vi "Create New File.vi"(8 "error in (no error)":errorcluster, 11 "[M] TDMS Save in":refnum<class "[M] TDMS Save.lvclass">) -> (0 "error out":errorcluster, 3 "[M] TDMS Save out":refnum<class "[M] TDMS Save.lvclass">)   [LabVIEW 2023, in "[M] TDMS Save.lvlib" / "[M] TDMS Save.lvclass"]
uses:
  [M] TDMS Save.lvclass
  [M] TDMS Save.lvclass/[M] TDMS Save.ctl
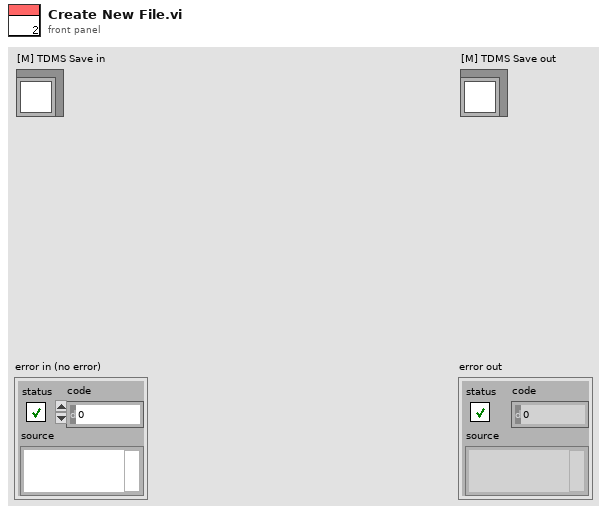
[diagram p1: front panel]
types:
  T1 = enum16{"open", "open or create", "create or replace", "create", "open (read-only)"}
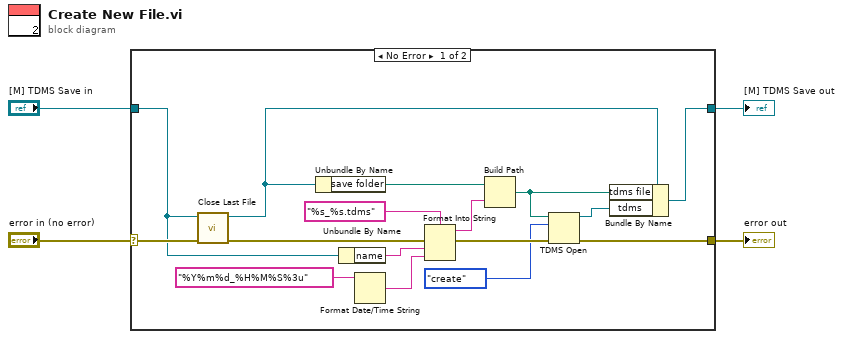
[diagram p0: block diagram]
diagram:
  n1 = case shown="No Error" "error in (no error)" {
    selector: "error in (no error)" -> [w20 w22]
    tunnel: [w9 w22] -> w3
    tunnel: [w8 w21] -> w1
    tunnel: "[M] TDMS Save in" -> [w12 w21]
    frame No Error {
      n2 = call "Close Last File.vi"("error in (no error)"=w20, "[M] TDMS Save in"=w12) -> ("error out"=w6:errorcluster, "[M] TDMS Save out"=w7:refnum<class "[M] TDMS Save.lvclass">)  [unwired: 8 in]
      n3 = Unbundle By Name(w7) -> ("save folder"=w15:path)
      n4 = Unbundle By Name(w12) -> ("name"=w18:string)
      n5 = Format Date/Time String(time format string (%c)="%Y%m%d_%H%M%S%3u") -> (date/time string=w17:string)  [unwired: 2 in]
      n6 = Format Into String(format string="%s_%s.tdms", error in=w6, w18, w17) -> (resulting string=w14:string, error out=w16:errorcluster)  [unwired: 1 in]
      n7 = Build Path(base path=w15, name or relative path=w14) -> (appended path=w11:path)
      n8 = TDMS Open(8:w16, 10:T1."create" ("operation (0:open)"), 11:w11) -> (0:w9:errorcluster, 3:w10:refnum<k34>)  [unwired: 4 in]
      n9 = Bundle By Name(cluster=w7, "tdms file"=w11, "tdms"=w10) -> (w8:refnum<class "[M] TDMS Save.lvclass">)
    }
    frame Error {
    }
  }
  "error out" <- w3
  "[M] TDMS Save out" <- w1
